vi "VariablesGlobales.vi"() -> ()   [LabVIEW 2020]
panel:
  in  "Panel_Color":T1
  out "Posicion_Galon":i32
  out "FIT 1":dbl
  out "B 1":bool
  out "Contador de Galones":dbl
  out "LSL 5":bool
  out "LSL 4":bool
  out "LSL 3":bool
  out "LSL 2":bool
  out "LSL 1":bool
  out "LSH 5":bool
  out "LSH 4":bool
  out "LSH 3":bool
  out "LSH 2":bool
  out "LSH 1":bool
  out "M1":bool
  out "FV 5":bool
  out "FV 4":bool
  out "FV 3":bool
  out "FV 2":bool
  out "FV 1":bool
  out "Mixer":bool
  out "Galón":bool
  out "Cilindro 2":bool
  out "Sellado":bool
  out "S 9":bool
  out "S 8":bool
  out "S 7":bool
  out "S 6":bool
  out "S 5":bool
  out "S 4":bool
  out "S 3":bool
  out "S 2":bool
  out "S 1":bool
  out "B 5":bool
  out "B 4":bool
  out "B 3":bool
  out "B 2":bool
  out "FIT 5":dbl
  out "FIT 4":dbl
  out "FIT 3":dbl
  out "FIT 2":dbl
  out "tk blanco":dbl(slide) scale=0.0..100.0
  out "tk negro":dbl(slide) scale=0.0..100.0
  out "tk azul":dbl(slide) scale=0.0..100.0
  out "tk amarillo":dbl(slide) scale=0.0..100.0
  out "tk rojo":dbl(slide) scale=0.0..100.0
  # "Yellow"
  # "Red"
  # "Blue"
  # "Black"
  # "White"
  # "gal"
  # "gal"
  # "gal"
  # "gal"
  # "gal"
  # "Etiquetado"
  # "Mezclado"
  # "gal"
  # "gal"
  # "gal"
  # "gal"
  # "Unidades"
  # "Panel de Selección de Color"
  # "gal"
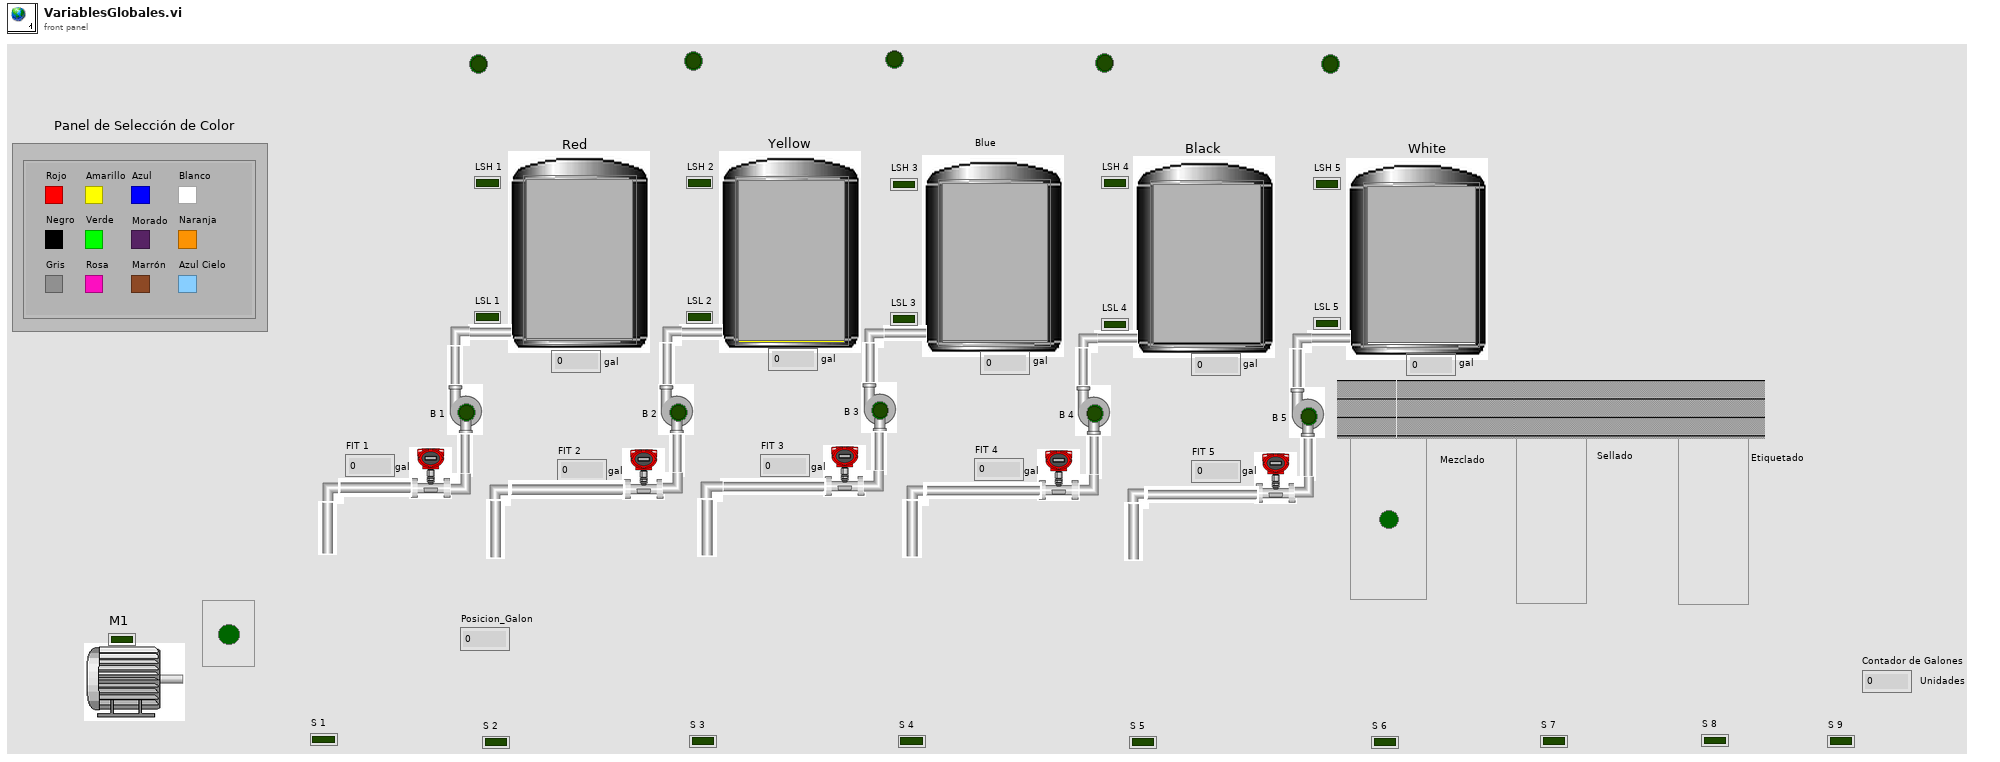
[diagram p1: front panel]
types:
  T1 = cluster{"Rojo":bool, "Amarillo":bool, "Azul":bool, "Blanco":bool, "Negro":bool, "Verde":bool, "Morado":bool, "Naranja":bool, "Gris":bool, "Rosa":bool, "Marrón ":bool, "Azul Cielo":bool}
diagram:
